vi "Configure Set Point.vi"(8 "error in (no error)":errorcluster, 10 "Set Point":T1, 11 "Temperature Control in":refnum<class "Temperature Control.lvclass">) -> (0 "error out":errorcluster, 3 "Temperature Control out":refnum<class "Temperature Control.lvclass">)   [LabVIEW 2020, in "Temperature Control.lvclass"]
uses:
  Temperature Control.lvclass
  Controls/Set point.ctl
  Temperature Control.lvclass/Temperature Control.ctl
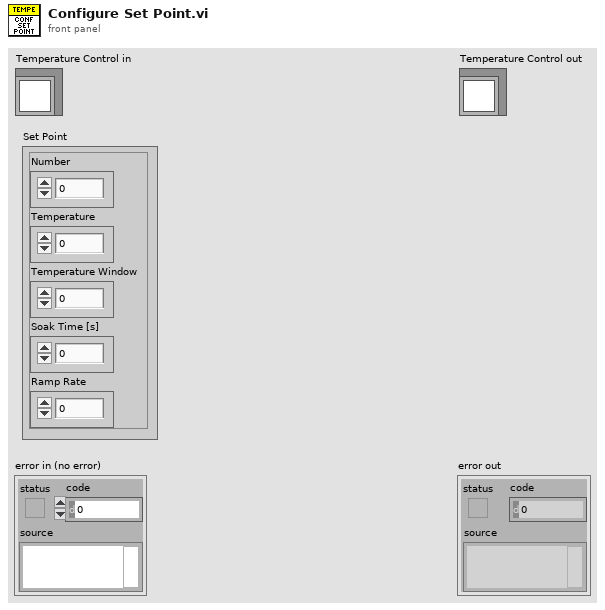
[diagram p1: front panel]
types:
  T1 = typedef "Temperature Control.lvclass/Set point.ctl" = cluster{"Number":u32, "Temperature":dbl, "Temperature Window":dbl, "Soak Time [s]":u32, "Ramp Rate":dbl}
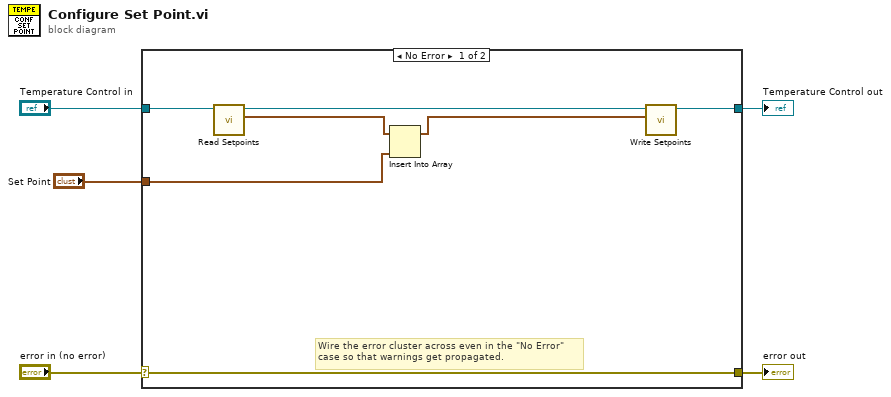
[diagram p0: block diagram]
diagram:
  n1 = case shown="No Error" "error in (no error)" {
    selector: "error in (no error)" -> [w12 w14]
    tunnel: [w12 w14] -> w4
    tunnel: [w10 w13] -> w2
    tunnel: "Temperature Control in" -> [w11 w13]
    tunnel: "Set Point" -> [w7 _]
    frame No Error {
      # "Wire the error cluster across even in the \"No Error\"\ncase so that warnings get propagated."
      n2 = call "Read Setpoints.vi"("Temperature Control in"=w11) -> ("Setpoints"=w8:T1[], "Temperature Control out"=w9:refnum<class "Temperature Control.lvclass">)  [unwired: 9 in]
      n3 = Insert Into Array(array=w8, new element=w7) -> (w6:T1[])  [unwired: 1 in]
      n4 = call "Write Setpoints.vi"("Setpoints"=w6, "Temperature Control in"=w9) -> ("Temperature Control out"=w10:refnum<class "Temperature Control.lvclass">)  [unwired: 9 in]
    }
    frame Error {
    }
  }
  "error out" <- w4
  "Temperature Control out" <- w2
